vi "drivetrain_raw_to_ftsec.vi"(11 "Drive Data":cluster{"Left":dbl, "Right":dbl}) -> (3 "Drive Data Out":cluster{"Left":dbl, "Right":dbl})   [LabVIEW 2011]
uses:
  drivetrain_globals.vi
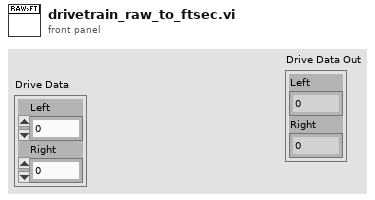
[diagram p1: front panel]
types:
  T1 = typedef "gear_shift_state.ctl" = enum16{"low", "high"}
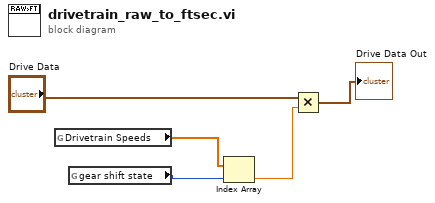
[diagram p0: block diagram]
diagram:
  n1 = global read "drivetrain_globals.vi" "Drivetrain Speeds"() -> (w5:dbl[])
  n2 = global read "drivetrain_globals.vi" "gear shift state"() -> (w1:T1)
  n3 = Index Array(array=w5, index=w1) -> (element=w2:dbl)
  n4 = Multiply(x="Drive Data", y=w2) -> (x*y=→"Drive Data Out":cluster{"Left":dbl, "Right":dbl})
